vi "fgv_ekf_motion-model.vi"(10 "u":T1, 11 "x_true":T1) -> (3 "x_true out":T1)   [LabVIEW 2019]
uses:
  <vilib>/Analysis/Matrix/Datatypes/RealMatrix.ctl
  Ctrl/cmd_common.ctl
  <vilib>/Analysis/baseanly.llb/Real A x B.vi
  <vilib>/Analysis/Matrix/Numeric/Add/Add - RM,RM.vi
  <vilib>/Analysis/Matrix/NI_Matrix.lvlib
  <vilib>/Analysis/NI_AALBase.lvlib
panel:
  out "B":T1
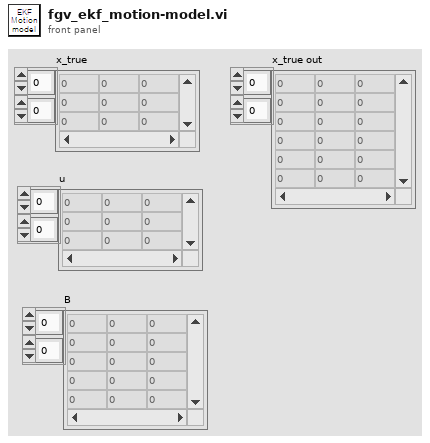
[diagram p1: front panel]
types:
  T1 = typedef "NI_Matrix.lvlib/RealMatrix.ctl" = dbl[][]
  T2 = typedef "cmd_common.ctl" = enum16{"read", "write"}
  T3 = cluster{"Q":T1, "R":T1, "input Noise":T1, "GPS noise":T1, "DT":dbl}
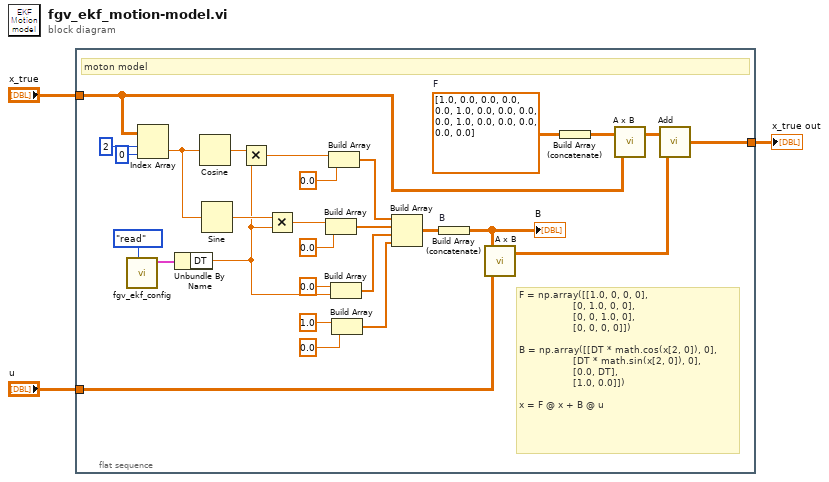
[diagram p0: block diagram]
diagram:
  n1 = flat-sequence {
    tunnel: "x_true" -> [w7]
    tunnel: "u" -> [w6]
    tunnel: [w9] -> w1
    frame #0 {
      w12 = dbl[][] [[1.0, 0.0, 0.0, 0.0], [0.0, 1.0, 0.0, 0.0], [0.0, 0.0, 1.0, 0.0], [0.0, 0.0, 0.0, 0.0]]  # F
      # "F = np.array([[1.0, 0, 0, 0],\n                  [0, 1.0, 0, 0],\n                  [0, 0, 1.0, 0],\n                  [0, 0, 0, 0]])\n\nB = np.array([[DT * math.cos(x[2, 0]), 0],\n                  [DT * math.sin(x[2, 0]), 0],\n                  [0.0, DT],\n                  [1.0, 0.0]])\n\nx = F @ x + B @ u"
      # "moton model"
      n2 = call "fgv_ekf_config.vi"("cmd"=cmd_common."read") -> ("set var out"=w5:T3)  [unwired: 10 in]
      n3 = Index Array(array=w7, index (row)=2 ("인덱스 (행)"), index (col)=0 ("인덱스 (열)")) -> (element=w27:dbl)
      n4 = Unbundle By Name(w5) -> ("DT"=w4:dbl)
      n5 = Cosine(x=w27) -> (cos(x)=w29:dbl)
      n6 = Sine(x=w27) -> (sin(x)=w28:dbl)
      n7 = Multiply(x=w29, y=w4) -> (x*y=w26:dbl)
      n8 = Multiply(x=w28, y=w4) -> (x*y=w23:dbl)
      n9 = Build Array(w23, 0.0 ("원소")) -> (w17:dbl[])
      n10 = Build Array(w26, 0.0 ("원소")) -> (w16:dbl[])
      n11 = Build Array(0.0 ("원소"), w4) -> (w18:dbl[])
      n12 = Build Array(1.0 ("원소"), 0.0 ("원소")) -> (w19:dbl[])
      n13 = Build Array(w16, w17, w18, w19) -> (w15:dbl[][])
      n14 = Build Array (concatenate) "B"(w15) -> (w14:T1)
      "B" <- w14
      n15 = call-poly <vilib>:"A x B.vi"("B"=w6, "A"=w14) -> ("A x B"=w13:T1)  [unwired: 1 out]
      n16 = Build Array (concatenate)(w12) -> (w8:T1)
      n17 = call-poly <vilib>:"A x B.vi"("B"=w7, "A"=w8) -> ("A x B"=w11:T1)  [unwired: 1 out]
      n18 = call-poly <vilib>:"Add.vi"("Real Matrix B"=w13, "Real Matrix A"=w11) -> ("A + B"=w9:T1)
    }
  }
  "x_true out" <- w1
